vi "Lang Set Menu.vi"(8 "error in (no error)":errorcluster, 10 "Menu":T1, 11 "LF2R IDE in":refnum<class "Main Panel.lvclass">) -> (0 "error out":errorcluster, 3 "LF2R IDE out":refnum<class "Main Panel.lvclass">)   [LabVIEW 2018, in "Main Panel.lvlib" / "Main Panel.lvclass"]
uses:
  Main Panel.lvclass
  Framework/Framework/Const Lang MainWnd Menu.ctl
  Framework/Framework/Const Lang Property.ctl
  Menu Item.ctl
  Main Panel.lvclass/Main Panel.ctl
  <userlib>/_MGI/Menu Building/MenuItem/MGI_MenuItem.lvclass
  Framework/Framework/Framework.lvclass
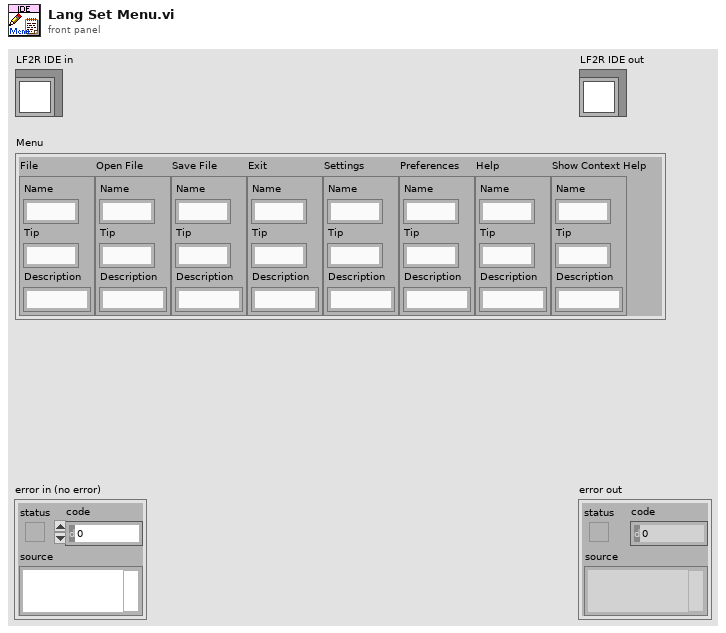
[diagram p1: front panel]
types:
  T1 = typedef "Framework.lvlib/Framework.lvclass/Const Lang MainWnd Menu.ctl" = cluster{"File":T2, "Open File":T2, "Save File":T2, "Exit":T2, "Settings":T2, "Preferences":T2, "Help":T2, "Show Context Help":T2}
  T2 = typedef "Framework.lvlib/Framework.lvclass/Const Lang Property.ctl" = cluster{"Name":string, "Tip":string, "Description":string}
  T3 = typedef "Main Panel.lvlib/Main Panel.lvclass/Menu Item.ctl" = enum16{"Invalid Item", "File", "Open File", "Save File", "Exit", "Settings", "Preferences", "Help", "Show Context Help"}
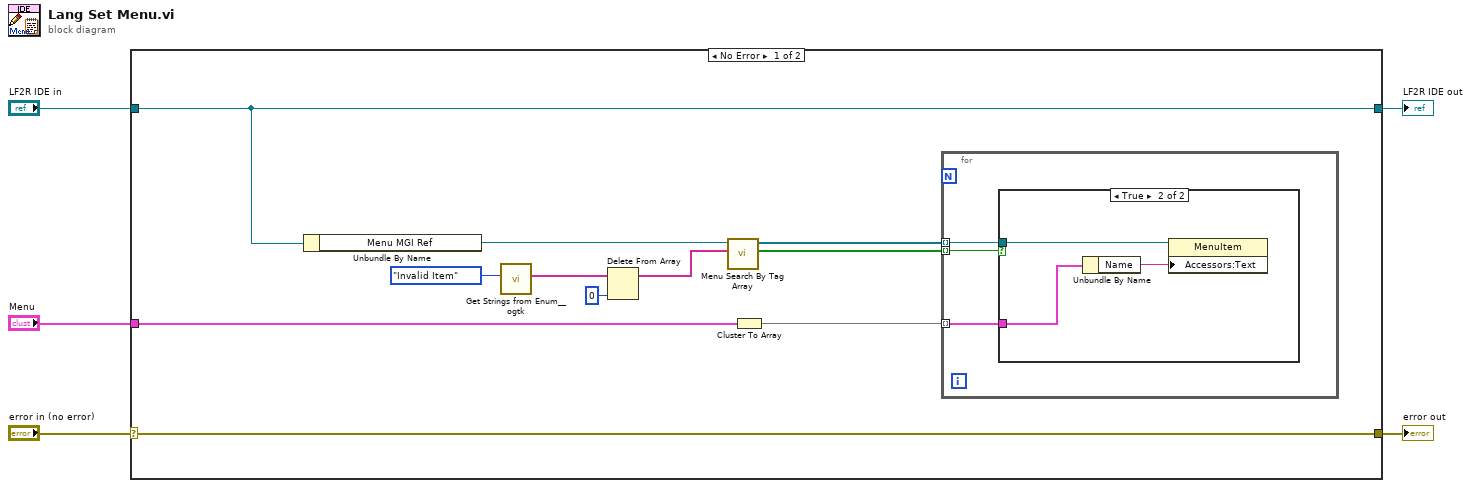
[diagram p0: block diagram]
diagram:
  n1 = case shown="No Error" "error in (no error)" {
    selector: "error in (no error)" -> [w14 w24]
    tunnel: [w14 w24] -> w4
    tunnel: [w16 w23] -> w2
    tunnel: "LF2R IDE in" -> [w16 w23]
    tunnel: "Menu" -> [w11 _]
    frame No Error {
      n2 = Unbundle By Name(w16) -> ("Menu MGI Ref"=w15:refnum<class "MGI_VI.lvclass">)
      n3 = call <userlib>:"Get Strings from Enum__ogtk.vi"("Enum"=Menu_Item."Invalid Item" ("Menu Item")) -> ("Enum Strings"=w8:string[])  [unwired: 7 in, 3 out]
      n4 = Delete From Array(array=w8, index=0) -> (array with subset deleted=w7:string[])  [unwired: 1 in, 1 out]
      n5 = call "Menu Search By Tag Array.vi"("Tag Array"=w7, "Menu MGI Ref"=w15) -> ("Found?"=w6:bool[], "Menu Item Array"=w12:refnum<data-value>[])  [unwired: 7 in, 1 out]
      n6 = Cluster To Array(cluster=w11) -> (array=w10:T2[])
      n7 = for {
        tunnel: w12 -> [w19] mode=indexing
        tunnel: w10 -> [w18] mode=indexing
        tunnel: w6 -> [w17] mode=indexing
        n8 = case shown="True" w17 {
          tunnel: w19 -> [_ w22]
          tunnel: w18 -> [_ w21]
          frame False {
          }
          frame True {
            n9 = Unbundle By Name(w21) -> ("Name"=w20:string)
            n10 = property class="MenuItem"(reference=w22, "Accessors:Text"=w20) -> ()  [unwired: 1 in, 2 out]
          }
        }
      }
    }
    frame Error {
    }
  }
  "error out" <- w4
  "LF2R IDE out" <- w2
